vi "REPORT.DIGIAL offset.vi"(9 "Vasic":i32, 10 "Config Test IN":T1={"Config HW"={"VISA Rigol DP832"="USB0::0x1AB1::0x0E11::DP8C191500901::INSTR", "Config Rigol DP832"=[{"Channel"=0, "V Limit"=5.5, "I Limit"=0.5, "V Out"=5.0}, {"Channel"=1, "V Limit"=5.5, "I Limit"=0.8, "V Out"=5.0}, {"Channel"=2, "V Limit"=5.5, "I Limit"=0.2, "V Out"=0.0}], "CTA Test#"="CTA013 A", "FT_Handle"=432866568, "Espera acceso FT"=10, "VISA Tek MDO3104"="Rigol_DP832", "VISA Key 81160A"="Rigol_DP832"}, "Config Test"=[{"Vasic"=2.8, "Global Reset"=FALSE, "Test Register?"=FALSE, "Test ADC?"=FALSE, "Test ADC"={"Repeats ADC"=100, "Max Desviation"=0.1}, "Limits ADC"={"Low"=[1.9, 1.3, 0.65, 0.0, 1.6, 1.4, 1.4, 0.9, 2.1, 0.85, 1.9], "High"=[2.1, 1.5, 0.85, 0.1, 1.4, 1.2, 1.2, 0.7, 1.9, 0.65, 1.7]}, "Test Max PN Min NP?"=FALSE, "Limits Max PN Min NP"={"Max P Upper"=2.177000045776367, "Min P Upper"=1.474, "Max N Upper"=1.475, "Min N Upper"=0.818, "Max P Lower"=1.888, "Min P Lower "=1.321, "Max N Lower"=1.322, "Min N Lower"=0.73}, "Test Rate Scan?"=FALSE, "Vin Rate Scan"=[], "Limits Rate Scan"={"High"=[0.15, 0.242, 0.331, 0.425, 0.512, 0.6, 0.688, 0.774, 0.847, 0.91], "Low"=[0.021, 0.11, 0.189, 0.27, 0.347, 0.421, 0.487, 0.551, 0.601, 0.635]}, "Test Rate Scan Adders?"=FALSE, "Vin Rate Adders"=[], "Limits Rate Scan adders"={"High"=[], "Low"=[]}, "Test offset analog?"=FALSE, "Lim Offset Analog"={"Max Analog"=0.05, "Min Analog"=-0.05}, "Test offset digital?"=FALSE, "Lim offset Dig"={"Max Dig"=0.05}, "Vasic real f.a."=2.8, "IBIAS"=FALSE, "VALUE IBIAS"=63}, {"Vasic"=2.8, "Global Reset"=FALSE, "Test Register?"=FALSE, "Test ADC?"=FALSE, "Test ADC"={"Repeats ADC"=100, "Max Desviation"=0.1}, "Limits ADC"={"Low"=[1.9, 1.3, 0.65, 0.0, 1.6, 1.4, 1.4, 0.9, 2.1, 0.85, 1.9], "High"=[2.1, 1.5, 0.85, 0.1, 1.4, 1.2, 1.2, 0.7, 1.9, 0.65, 1.7]}, "Test Max PN Min NP?"=FALSE, "Limits Max PN Min NP"={"Max P Upper"=2.177000045776367, "Min P Upper"=1.474, "Max N Upper"=1.475, "Min N Upper"=0.818, "Max P Lower"=1.888, "Min P Lower "=1.321, "Max N Lower"=1.322, "Min N Lower"=0.73}, "Test Rate Scan?"=FALSE, "Vin Rate Scan"=[], "Limits Rate Scan"={"High"=[0.15, 0.242, 0.331, 0.425, 0.512, 0.6, 0.688, 0.774, 0.847, 0.91], "Low"=[0.021, 0.11, 0.189, 0.27, 0.347, 0.421, 0.487, 0.551, 0.601, 0.635]}, "Test Rate Scan Adders?"=FALSE, "Vin Rate Adders"=[], "Limits Rate Scan adders"={"High"=[], "Low"=[]}, "Test offset analog?"=FALSE, "Lim Offset Analog"={"Max Analog"=0.05, "Min Analog"=-0.05}, "Test offset digital?"=FALSE, "Lim offset Dig"={"Max Dig"=0.05}, "Vasic real f.a."=2.8, "IBIAS"=FALSE, "VALUE IBIAS"=63}, {"Vasic"=2.8, "Global Reset"=FALSE, "Test Register?"=FALSE, "Test ADC?"=FALSE, "Test ADC"={"Repeats ADC"=100, "Max Desviation"=0.1}, "Limits ADC"={"Low"=[1.9, 1.3, 0.65, 0.0, 1.6, 1.4, 1.4, 0.9, 2.1, 0.85, 1.9], "High"=[2.1, 1.5, 0.85, 0.1, 1.4, 1.2, 1.2, 0.7, 1.9, 0.65, 1.7]}, "Test Max PN Min NP?"=FALSE, "Limits Max PN Min NP"={"Max P Upper"=2.177000045776367, "Min P Upper"=1.474, "Max N Upper"=1.475, "Min N Upper"=0.818, "Max P Lower"=1.888, "Min P Lower "=1.321, "Max N Lower"=1.322, "Min N Lower"=0.73}, "Test Rate Scan?"=FALSE, "Vin Rate Scan"=[], "Limits Rate Scan"={"High"=[0.15, 0.242, 0.331, 0.425, 0.512, 0.6, 0.688, 0.774, 0.847, 0.91], "Low"=[0.021, 0.11, 0.189, 0.27, 0.347, 0.421, 0.487, 0.551, 0.601, 0.635]}, "Test Rate Scan Adders?"=FALSE, "Vin Rate Adders"=[], "Limits Rate Scan adders"={"High"=[], "Low"=[]}, "Test offset analog?"=FALSE, "Lim Offset Analog"={"Max Analog"=0.05, "Min Analog"=-0.05}, "Test offset digital?"=FALSE, "Lim offset Dig"={"Max Dig"=0.05}, "Vasic real f.a."=2.8, "IBIAS"=FALSE, "VALUE IBIAS"=63}, {"Vasic"=2.8, "Global Reset"=FALSE, "Test Register?"=FALSE, "Test ADC?"=FALSE, "Test ADC"={"Repeats ADC"=100, "Max Desviation"=0.1}, "Limits ADC"={"Low"=[1.9, 1.3, 0.65, 0.0, 1.6, 1.4, 1.4, 0.9, 2.1, 0.85, 1.9], "High"=[2.1, 1.5, 0.85, 0.1, 1.4, 1.2, 1.2, 0.7, 1.9, 0.65, 1.7]}, "Test Max PN Min NP?"=FALSE, "Limits Max PN Min NP"={"Max P Upper"=2.177000045776367, "Min P Upper"=1.474, "Max N Upper"=1.475, "Min N Upper"=0.818, "Max P Lower"=1.888, "Min P Lower "=1.321, "Max N Lower"=1.322, "Min N Lower"=0.73}, "Test Rate Scan?"=FALSE, "Vin Rate Scan"=[], "Limits Rate Scan"={"High"=[0.15, 0.242, 0.331, 0.425, 0.512, 0.6, 0.688, 0.774, 0.847, 0.91], "Low"=[0.021, 0.11, 0.189, 0.27, 0.347, 0.421, 0.487, 0.551, 0.601, 0.635]}, "Test Rate Scan Adders?"=FALSE, "Vin Rate Adders"=[], "Limits Rate Scan adders"={"High"=[], "Low"=[]}, "Test offset analog?"=FALSE, "Lim Offset Analog"={"Max Analog"=0.05, "Min Analog"=-0.05}, "Test offset digital?"=FALSE, "Lim offset Dig"={"Max Dig"=0.05}, "Vasic real f.a."=2.8, "IBIAS"=FALSE, "VALUE IBIAS"=63}], "Result"=[{"Vasic Volt"=0, "Test Registros"={"Default Register OK"=FALSE, "Pattern Default"=[], "Read Default"=[], "W/R Register OK"=FALSE, "Pattern W/R"=[], "Read W/R"=[]}, "Test Dacs"={"Desviacion OK"=FALSE, "Means"=[], "Deviations"=[], "Desviations OK"=[], "Means OK"=[], "Graph Histogram"=[]}, "Test Max-Min PN"={"Max P Mini N OK"=FALSE, "PTHT Max P Min N"=[], "PTHT Max P Min N OK"=[], "NTHT Max P Min N"=[], "NTHT Max P Min N OK"=[], "Min P Max N OK"=FALSE, "PTHT Max N Min P"=[], "PTHT Max N Min P OK"=[], "NTHT Max N Min P"=[], "NTHT Max N Min P OK"=[], "Ref"=[]}, "Test Rate Scan"={"Rate Scan OK"=FALSE, "DAC TH0,TH1,TH2"=[], "Volt HLTH"=[], "Rate HLTH OK"=[], "DAC TH3,TH4,TH5"=[], "Volt LLTH"=[], "Rate LLTH 2 OK"=[], "Scaler 0"=[], "Ref"=[], "OFFSET HLTH"=[], "OFFSET LLTH"=[], "Real Voltage"=[]}, "Test Rate Scan adders"={"Rate Scan Adders OK"=FALSE, "DAC TH0,TH1,TH2"=[], "Volt HLTH"=[], "Add HLTH OK"=[], "DAC TH3,TH4,TH5"=[], "Volt LLTH"=[], "Add LLTH 2 OK"=[], "Scaler 0"=[], "Ref"=[], "OFFSET HLTH"=[], "OFFSET LLTH"=[], "Real Voltage"=[]}, "Test Offset Analog"={"Offset Analog OK"=FALSE, "V ADDOUT"=[], "Offset OK"=[], "Ref"=[]}, "Test Offset Digital"={"Offset Digital OK"=FALSE, "SCALER 1 START"=[], "SCALER 1 STOP"=[], "THX START"=[], "THX STOP"=[], "VHLTH START"=[], "VHLTH STOP"=[], "Index 1 Start"=[], "index 1 Stop"=[], "SCALER 2 START"=[], "SCALER 2 STOP"=[], "THX+3 START"=[], "THX+3 STOP"=[], "VLLTH START"=[], "VLLTH STOP"=[], "Index 2 Start"=[], "index 2 Stop"=[], "Dig HLTH OK"=[], "Dig LLTH 2 OK"=[], "Ref"=[]}, "info hardware"={"Iout V1"=0.0, "Iout V2"=0.0, "Iout V3"=0.0, "Vout V1"=0.0, "Vout V2"=0.0, "Vout V3"=0.0, "Temp"=0.0}, "Test Offset Analog add"={"Offset Analog add OK"=FALSE, "V ADDOUT add"=[], "Offset add OK"=[], "Ref add"=[]}, "info temp"={"T Asic Registers"=0.0, "T Board Test. ADC"=0.0, "T Asic Max Min N P"=0.0, "T Adc count"=0.0, "T Asic Digital Offset"=0.0, "T Asic Analog Offset"=0.0, "T Asic Analog add"=0.0, "T Asic Rate Scan"=0.0, "T Asic Rate Scan Adders"=0.0, "T Final"=0.0}}, {"Vasic Volt"=0, "Test Registros"={"Default Register OK"=FALSE, "Pattern Default"=[], "Read Default"=[], "W/R Register OK"=FALSE, "Pattern W/R"=[], "Read W/R"=[]}, "Test Dacs"={"Desviacion OK"=FALSE, "Means"=[], "Deviations"=[], "Desviations OK"=[], "Means OK"=[], "Graph Histogram"=[]}, "Test Max-Min PN"={"Max P Mini N OK"=FALSE, "PTHT Max P Min N"=[], "PTHT Max P Min N OK"=[], "NTHT Max P Min N"=[], "NTHT Max P Min N OK"=[], "Min P Max N OK"=FALSE, "PTHT Max N Min P"=[], "PTHT Max N Min P OK"=[], "NTHT Max N Min P"=[], "NTHT Max N Min P OK"=[], "Ref"=[]}, "Test Rate Scan"={"Rate Scan OK"=FALSE, "DAC TH0,TH1,TH2"=[], "Volt HLTH"=[], "Rate HLTH OK"=[], "DAC TH3,TH4,TH5"=[], "Volt LLTH"=[], "Rate LLTH 2 OK"=[], "Scaler 0"=[], "Ref"=[], "OFFSET HLTH"=[], "OFFSET LLTH"=[], "Real Voltage"=[]}, "Test Rate Scan adders"={"Rate Scan Adders OK"=FALSE, "DAC TH0,TH1,TH2"=[], "Volt HLTH"=[], "Add HLTH OK"=[], "DAC TH3,TH4,TH5"=[], "Volt LLTH"=[], "Add LLTH 2 OK"=[], "Scaler 0"=[], "Ref"=[], "OFFSET HLTH"=[], "OFFSET LLTH"=[], "Real Voltage"=[]}, "Test Offset Analog"={"Offset Analog OK"=FALSE, "V ADDOUT"=[], "Offset OK"=[], "Ref"=[]}, "Test Offset Digital"={"Offset Digital OK"=FALSE, "SCALER 1 START"=[], "SCALER 1 STOP"=[], "THX START"=[], "THX STOP"=[], "VHLTH START"=[], "VHLTH STOP"=[], "Index 1 Start"=[], "index 1 Stop"=[], "SCALER 2 START"=[], "SCALER 2 STOP"=[], "THX+3 START"=[], "THX+3 STOP"=[], "VLLTH START"=[], "VLLTH STOP"=[], "Index 2 Start"=[], "index 2 Stop"=[], "Dig HLTH OK"=[], "Dig LLTH 2 OK"=[], "Ref"=[]}, "info hardware"={"Iout V1"=0.0, "Iout V2"=0.0, "Iout V3"=0.0, "Vout V1"=0.0, "Vout V2"=0.0, "Vout V3"=0.0, "Temp"=0.0}, "Test Offset Analog add"={"Offset Analog add OK"=FALSE, "V ADDOUT add"=[], "Offset add OK"=[], "Ref add"=[]}, "info temp"={"T Asic Registers"=0.0, "T Board Test. ADC"=0.0, "T Asic Max Min N P"=0.0, "T Adc count"=0.0, "T Asic Digital Offset"=0.0, "T Asic Analog Offset"=0.0, "T Asic Analog add"=0.0, "T Asic Rate Scan"=0.0, "T Asic Rate Scan Adders"=0.0, "T Final"=0.0}}, {"Vasic Volt"=0, "Test Registros"={"Default Register OK"=FALSE, "Pattern Default"=[], "Read Default"=[], "W/R Register OK"=FALSE, "Pattern W/R"=[], "Read W/R"=[]}, "Test Dacs"={"Desviacion OK"=FALSE, "Means"=[], "Deviations"=[], "Desviations OK"=[], "Means OK"=[], "Graph Histogram"=[]}, "Test Max-Min PN"={"Max P Mini N OK"=FALSE, "PTHT Max P Min N"=[], "PTHT Max P Min N OK"=[], "NTHT Max P Min N"=[], "NTHT Max P Min N OK"=[], "Min P Max N OK"=FALSE, "PTHT Max N Min P"=[], "PTHT Max N Min P OK"=[], "NTHT Max N Min P"=[], "NTHT Max N Min P OK"=[], "Ref"=[]}, "Test Rate Scan"={"Rate Scan OK"=FALSE, "DAC TH0,TH1,TH2"=[], "Volt HLTH"=[], "Rate HLTH OK"=[], "DAC TH3,TH4,TH5"=[], "Volt LLTH"=[], "Rate LLTH 2 OK"=[], "Scaler 0"=[], "Ref"=[], "OFFSET HLTH"=[], "OFFSET LLTH"=[], "Real Voltage"=[]}, "Test Rate Scan adders"={"Rate Scan Adders OK"=FALSE, "DAC TH0,TH1,TH2"=[], "Volt HLTH"=[], "Add HLTH OK"=[], "DAC TH3,TH4,TH5"=[], "Volt LLTH"=[], "Add LLTH 2 OK"=[], "Scaler 0"=[], "Ref"=[], "OFFSET HLTH"=[], "OFFSET LLTH"=[], "Real Voltage"=[]}, "Test Offset Analog"={"Offset Analog OK"=FALSE, "V ADDOUT"=[], "Offset OK"=[], "Ref"=[]}, "Test Offset Digital"={"Offset Digital OK"=FALSE, "SCALER 1 START"=[], "SCALER 1 STOP"=[], "THX START"=[], "THX STOP"=[], "VHLTH START"=[], "VHLTH STOP"=[], "Index 1 Start"=[], "index 1 Stop"=[], "SCALER 2 START"=[], "SCALER 2 STOP"=[], "THX+3 START"=[], "THX+3 STOP"=[], "VLLTH START"=[], "VLLTH STOP"=[], "Index 2 Start"=[], "index 2 Stop"=[], "Dig HLTH OK"=[], "Dig LLTH 2 OK"=[], "Ref"=[]}, "info hardware"={"Iout V1"=0.0, "Iout V2"=0.0, "Iout V3"=0.0, "Vout V1"=0.0, "Vout V2"=0.0, "Vout V3"=0.0, "Temp"=0.0}, "Test Offset Analog add"={"Offset Analog add OK"=FALSE, "V ADDOUT add"=[], "Offset add OK"=[], "Ref add"=[]}, "info temp"={"T Asic Registers"=0.0, "T Board Test. ADC"=0.0, "T Asic Max Min N P"=0.0, "T Adc count"=0.0, "T Asic Digital Offset"=0.0, "T Asic Analog Offset"=0.0, "T Asic Analog add"=0.0, "T Asic Rate Scan"=0.0, "T Asic Rate Scan Adders"=0.0, "T Final"=0.0}}, {"Vasic Volt"=0, "Test Registros"={"Default Register OK"=FALSE, "Pattern Default"=[], "Read Default"=[], "W/R Register OK"=FALSE, "Pattern W/R"=[], "Read W/R"=[]}, "Test Dacs"={"Desviacion OK"=FALSE, "Means"=[], "Deviations"=[], "Desviations OK"=[], "Means OK"=[], "Graph Histogram"=[]}, "Test Max-Min PN"={"Max P Mini N OK"=FALSE, "PTHT Max P Min N"=[], "PTHT Max P Min N OK"=[], "NTHT Max P Min N"=[], "NTHT Max P Min N OK"=[], "Min P Max N OK"=FALSE, "PTHT Max N Min P"=[], "PTHT Max N Min P OK"=[], "NTHT Max N Min P"=[], "NTHT Max N Min P OK"=[], "Ref"=[]}, "Test Rate Scan"={"Rate Scan OK"=FALSE, "DAC TH0,TH1,TH2"=[], "Volt HLTH"=[], "Rate HLTH OK"=[], "DAC TH3,TH4,TH5"=[], "Volt LLTH"=[], "Rate LLTH 2 OK"=[], "Scaler 0"=[], "Ref"=[], "OFFSET HLTH"=[], "OFFSET LLTH"=[], "Real Voltage"=[]}, "Test Rate Scan adders"={"Rate Scan Adders OK"=FALSE, "DAC TH0,TH1,TH2"=[], "Volt HLTH"=[], "Add HLTH OK"=[], "DAC TH3,TH4,TH5"=[], "Volt LLTH"=[], "Add LLTH 2 OK"=[], "Scaler 0"=[], "Ref"=[], "OFFSET HLTH"=[], "OFFSET LLTH"=[], "Real Voltage"=[]}, "Test Offset Analog"={"Offset Analog OK"=FALSE, "V ADDOUT"=[], "Offset OK"=[], "Ref"=[]}, "Test Offset Digital"={"Offset Digital OK"=FALSE, "SCALER 1 START"=[], "SCALER 1 STOP"=[], "THX START"=[], "THX STOP"=[], "VHLTH START"=[], "VHLTH STOP"=[], "Index 1 Start"=[], "index 1 Stop"=[], "SCALER 2 START"=[], "SCALER 2 STOP"=[], "THX+3 START"=[], "THX+3 STOP"=[], "VLLTH START"=[], "VLLTH STOP"=[], "Index 2 Start"=[], "index 2 Stop"=[], "Dig HLTH OK"=[], "Dig LLTH 2 OK"=[], "Ref"=[]}, "info hardware"={"Iout V1"=0.0, "Iout V2"=0.0, "Iout V3"=0.0, "Vout V1"=0.0, "Vout V2"=0.0, "Vout V3"=0.0, "Temp"=0.0}, "Test Offset Analog add"={"Offset Analog add OK"=FALSE, "V ADDOUT add"=[], "Offset add OK"=[], "Ref add"=[]}, "info temp"={"T Asic Registers"=0.0, "T Board Test. ADC"=0.0, "T Asic Max Min N P"=0.0, "T Adc count"=0.0, "T Asic Digital Offset"=0.0, "T Asic Analog Offset"=0.0, "T Asic Analog add"=0.0, "T Asic Rate Scan"=0.0, "T Asic Rate Scan Adders"=0.0, "T Final"=0.0}}], "Execucion Test"={"Vasic Actual"=0}, "Config VGA"={"Theoretical Voltage"=[0.1, 0.2, 0.3, 0.4, 0.5, 0.6, 0.7, 0.8, 0.9, 1.0], "Real Voltage"=[0.10285, 0.20714, 0.29957, 0.40485, 0.49571, 0.60685, 0.69771, 0.80114, 0.89714, 0.99885], "Pulse Width"=57344, "Frecuency Pulse"=1000000.0, "VGA Gain"=[9, 16, 24, 34, 43, 52, 61, 72, 81, 93]}, "Test Info"={"Asic"="", "Operator"="", "Place"="", "Time start"=timestamp(0 s since 1904-01-01), "Time stop"=timestamp(0 s since 1904-01-01)}, "Info machine"={"SO"="", "SO Name"="", "SO Ver"="", "SO Build"="", "CPU"="", "APP"="", "APP YEAR"="", "APP ver"="", "APP User"="", "APP Serail"="", "MAC"=[], "PC NAME"=[], "PC IP"=[], "BIOS MANU"="", "BIOS NAME"="", "BIOS SERIAL"="", "BOARD MANU"="", "BOARD NAME"="", "BOARD SERIAL"="", "Driver Version"="", "Library Version"="", "FPGA Ver"=0, "ID CTA board"=0, "LAST BOOT"="", "LABVIEW Ver"=0}, "Partial Report"="", "CONFIG GEN"=[]} {"CONFIG GEN"."Vasic Theorical" min=1.0 max=1000000.0 step=1.0 format="%#_6pV"; "CONFIG GEN"."Frequency" min=0.001 max=333000000.0 step=1000.0 format="%#_6pHz"; "CONFIG GEN"."Leading Edge Time" min=1e-09 max=1.0 step=1e-10 format="%#_6ps"; "CONFIG GEN"."Trailing Edge Time" min=1e-09 max=1.0 step=1e-10 format="%#_6ps"; "CONFIG GEN"."Delay" min=0.0 max=1.0 step=1e-12 format="%#_6ps"; "CONFIG GEN"."Trigger Level Sync" items=["ECL", "TTL"]; "CONFIG GEN"."Trigger Sync Out" items=["AB"=3, "B"=2, "A"=1, "None"=0]; "CONFIG GEN"."Load" min=1.0 max=1000000.0 step=1.0 format="%#_6p"; "CONFIG GEN"."DC Offset" min=-10.0 max=10.0 step=0.1 format="%#_6pV"; "CONFIG GEN"."Amplitude" min=0.05 max=5.0 step=0.001 format="%#_6pV"; "CONFIG GEN"."Width Time" min=1.5e-09 max=1.0 step=1e-10 format="%#_6ps"; "CONFIG GEN"."Channel" items=["Channel1"=1, "Channel2"=2]; "Config VGA"."Theoretical Voltage" format="%1.4f"; "Config VGA"."VGA Gain" format="%02x"; "Config VGA"."Frecuency Pulse" format="%0_2p"; "Config VGA"."Pulse Width" format="%04x"; "Config VGA"."Real Voltage" format="%1.5f"; "Config Test"."VALUE IBIAS" max=63 step=1; "Config Test"."Vasic real f.a." min=2.8 max=3.8 step=0.01 format="%.2g"; "Config Test"."Limits Rate Scan adders"."Low" format="%1.3f"; "Config Test"."Limits Rate Scan adders"."High" format="%1.3f"; "Config Test"."Limits ADC"."High" format="%1.4f"; "Config Test"."Limits ADC"."Low" format="%1.3f"; "Config Test"."Lim offset Dig"."Max Dig" format="%.3g"; "Config Test"."Lim Offset Analog"."Min Analog" format="%.3g"; "Config Test"."Lim Offset Analog"."Max Analog" format="%.3g"; "Config Test"."Limits Rate Scan"."Low" format="%1.4f"; "Config Test"."Limits Rate Scan"."High" format="%1.3f"; "Config Test"."Limits Max PN Min NP"."Min P Upper" format="%.3g"; "Config Test"."Limits Max PN Min NP"."Min P Lower" format="%.3g"; "Config Test"."Limits Max PN Min NP"."Max N Lower" format="%.3g"; "Config Test"."Limits Max PN Min NP"."Max N Upper" format="%.3g"; "Config Test"."Limits Max PN Min NP"."Min N Lower" format="%.3g"; "Config Test"."Limits Max PN Min NP"."Min N Upper" format="%.3g"; "Config Test"."Limits Max PN Min NP"."Max P Upper" format="%.3g"; "Config Test"."Limits Max PN Min NP"."Max P Lower" format="%.3g"; "Config Test"."Vasic" min=2.8 max=3.8 step=0.01 format="%.2g"; "Config HW"."Config Rigol DP832"."Channel" items=["+30V Channel 1", "+30V Channel 2", "+5V Channel 3"]; "Config HW"."Config Rigol DP832"."V Limit" format="%.1g"; "Config HW"."Config Rigol DP832"."I Limit" format="%.1g"; "Config HW"."Config Rigol DP832"."V Out" format="%.1g"; "Result"."Test Registros"."Read W/R" format="%04x"; "Result"."Test Registros"."Pattern W/R" format="%04x"; "Result"."Test Registros"."Read Default" format="%04x"; "Result"."Test Registros"."Pattern Default" format="%04x"}, 11 "Text In":string) -> (3 "Text Out":string)   [LabVIEW 2019]
uses:
  Test.ctl
  TEST.TEST CONFIG HW.ctl
  Rigol DP832/DP832_Control Channels.ctl
  TEST.TEST CONFIG TEST MATRIZ.ctl
  TEST.TEST CONFIG TEST.ctl
  TEST.TEST RESULT.ctl
  test_result fvasic.ctl
  TEST.TEST EXECUTION TEST.ctl
  TEST.TEST CONFIG VGA.ctl
  TEST.TEST TEST INFO.ctl
  TEST.TEST INFO PC.ctl
  GenPulse_configurar.ctl
panel:
  # "Modo 2\nModo 3\nModo 4\nModo 2\nModo 3\nModo 4"
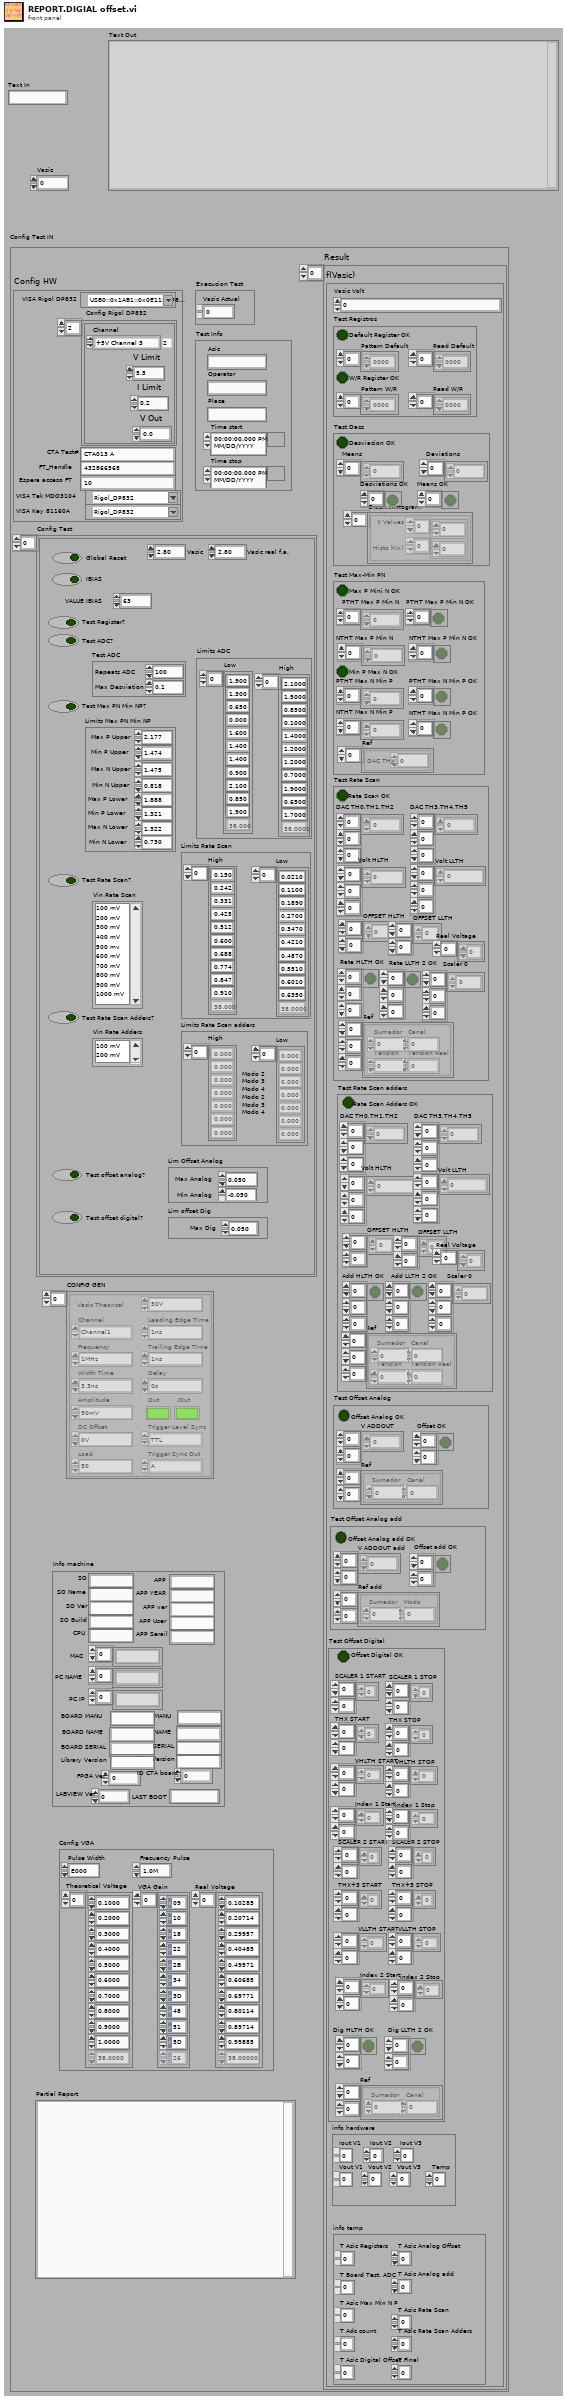
[diagram p1: front panel]
types:
  T1 = typedef "Test.ctl" = cluster{"Config HW":T2, "Config Test":T4, "Result":T6, "Execucion Test":T8, "Config VGA":T9, "Test Info":T10, "Info machine":T11, "Partial Report":string, "CONFIG GEN":T12[]}
  T2 = typedef "TEST.TEST CONFIG HW.ctl" = cluster{"VISA Rigol DP832":refnum<visa-resource-name>, "Config Rigol DP832":cluster{"Channel":T3, "V Limit":dbl, "I Limit":dbl, "V Out":dbl}[], "CTA Test#":string, "FT_Handle":u32, "Espera acceso FT":u32, "VISA Tek MDO3104":refnum<visa-resource-name>, "VISA Key 81160A":refnum<visa-resource-name>}
  T3 = typedef "DP832_Control Channels.ctl" = i32
  T4 = typedef "TEST.TEST CONFIG TEST MATRIZ.ctl" = T5[]
  T5 = typedef "TEST.TEST CONFIG TEST.ctl" = cluster{"Vasic":dbl, "Global Reset":bool, "Test Register?":bool, "Test ADC?":bool, "Test ADC":cluster{"Repeats ADC":i32, "Max Desviation":dbl}, "Limits ADC":cluster{"Low":dbl[], "High":dbl[]}, "Test Max PN Min NP?":bool, "Limits Max PN Min NP":cluster{"Max P Upper":dbl, "Min P Upper":dbl, "Max N Upper":dbl, "Min N Upper":dbl, "Max P Lower":dbl, "Min P Lower ":dbl, "Max N Lower":dbl, "Min N Lower":dbl}, "Test Rate Scan?":bool, "Vin Rate Scan":i32[], "Limits Rate Scan":cluster{"High":dbl[], "Low":dbl[]}, "Test Rate Scan Adders?":bool, "Vin Rate Adders":i32[], "Limits Rate Scan adders":cluster{"High":dbl[], "Low":dbl[]}, "Test offset analog?":bool, "Lim Offset Analog":cluster{"Max Analog":dbl, "Min Analog":dbl}, "Test offset digital?":bool, "Lim offset Dig":cluster{"Max Dig":dbl}, "Vasic real f.a.":dbl, "IBIAS":bool, "VALUE IBIAS":u8}
  T6 = typedef "TEST.TEST RESULT.ctl" = T7[]
  T7 = typedef "test_result fvasic.ctl" = cluster{"Vasic Volt":i32, "Test Registros":cluster{"Default Register OK":bool, "Pattern Default":u16[], "Read Default":u16[], "W/R Register OK":bool, "Pattern W/R":u16[], "Read W/R":u16[]}, "Test Dacs":cluster{"Desviacion OK":bool, "Means":dbl[], "Deviations":dbl[], "Desviations OK":bool[], "Means OK":bool[], "Graph Histogram":cluster{"X Values":dbl[], "Histo h(x)":i32[]}[]}, "Test Max-Min PN":cluster{"Max P Mini N OK":bool, "PTHT Max P Min N":dbl[], "PTHT Max P Min N OK":bool[], "NTHT Max P Min N":dbl[], "NTHT Max P Min N OK":bool[], "Min P Max N OK":bool, "PTHT Max N Min P":dbl[], "PTHT Max N Min P OK":bool[], "NTHT Max N Min P":dbl[], "NTHT Max N Min P OK":bool[], "Ref":cluster{"DAC THx":u8}[]}, "Test Rate Scan":cluster{"Rate Scan OK":bool, "DAC TH0,TH1,TH2":u16[][][], "Volt HLTH":dbl[][][], "Rate HLTH OK":bool[][][], "DAC TH3,TH4,TH5":u16[][][], "Volt LLTH":dbl[][][], "Rate LLTH 2 OK":bool[][][], "Scaler 0":u16[][][], "Ref":cluster{"Sumador":u8, "Canal":u8, "Tension":u8, "Tension Real":dbl}[][][], "OFFSET HLTH":dbl[][], "OFFSET LLTH":dbl[][], "Real Voltage":dbl[]}, "Test Rate Scan adders":cluster{"Rate Scan Adders OK":bool, "DAC TH0,TH1,TH2":u16[][][], "Volt HLTH":dbl[][][], "Add HLTH OK":bool[][][], "DAC TH3,TH4,TH5":u16[][][], "Volt LLTH":dbl[][][], "Add LLTH 2 OK":bool[][][], "Scaler 0":u16[][][], "Ref":cluster{"Sumador":u8, "Canal":u8, "Tension":u8, "Tension Real":dbl}[][][], "OFFSET HLTH":dbl[][], "OFFSET LLTH":dbl[][], "Real Voltage":dbl[]}, "Test Offset Analog":cluster{"Offset Analog OK":bool, "V ADDOUT":dbl[][], "Offset OK":bool[][], "Ref":cluster{"Sumador":u8, "Canal":u8}[][]}, "Test Offset Digital":cluster{"Offset Digital OK":bool, "SCALER 1 START":u16[][], "SCALER 1 STOP":u16[][], "THX START":u16[][], "THX STOP":u16[][], "VHLTH START":dbl[][], "VHLTH STOP":dbl[][], "Index 1 Start":i32[][], "index 1 Stop":i32[][], "SCALER 2 START":u16[][], "SCALER 2 STOP":u16[][], "THX+3 START":u16[][], "THX+3 STOP":u16[][], "VLLTH START":dbl[][], "VLLTH STOP":dbl[][], "Index 2 Start":i32[][], "index 2 Stop":i32[][], "Dig HLTH OK":bool[][], "Dig LLTH 2 OK":bool[][], "Ref":cluster{"Sumador":u8, "Canal":u8}[][]}, "info hardware":cluster{"Iout V1":dbl, "Iout V2":dbl, "Iout V3":dbl, "Vout V1":dbl, "Vout V2":dbl, "Vout V3":dbl, "Temp":dbl}, "Test Offset Analog add":cluster{"Offset Analog add OK":bool, "V ADDOUT add":dbl[][], "Offset add OK":bool[][], "Ref add":cluster{"Sumador":u8, "Modo":u8}[][]}, "info temp":cluster{"T Asic Registers":dbl, "T Board Test. ADC":dbl, "T Asic Max Min N P":dbl, "T Adc count":dbl, "T Asic Digital Offset":dbl, "T Asic Analog Offset":dbl, "T Asic Analog add":dbl, "T Asic Rate Scan":dbl, "T Asic Rate Scan Adders":dbl, "T Final":dbl}}
  T8 = typedef "TEST.TEST EXECUTION TEST.ctl" = cluster{"Vasic Actual":i32}
  T9 = typedef "TEST.TEST CONFIG VGA.ctl" = cluster{"Theoretical Voltage":dbl[], "Real Voltage":dbl[], "Pulse Width":u16, "Frecuency Pulse":dbl, "VGA Gain":u8[]}
  T10 = typedef "TEST.TEST TEST INFO.ctl" = cluster{"Asic":string, "Operator":string, "Place":string, "Time start":timestamp, "Time stop":timestamp}
  T11 = typedef "TEST.TEST INFO PC.ctl" = cluster{"SO":string, "SO Name":string, "SO Ver":string, "SO Build":string, "CPU":string, "APP":string, "APP YEAR":string, "APP ver":string, "APP User":string, "APP Serail":string, "MAC":string[], "PC NAME":string[], "PC IP":string[], "BIOS MANU":string, "BIOS NAME":string, "BIOS SERIAL":string, "BOARD MANU":string, "BOARD NAME":string, "BOARD SERIAL":string, "Driver Version":string, "Library Version":string, "FPGA Ver":u8, "ID CTA board":u64, "LAST BOOT":string, "LABVIEW Ver":u32}
  T12 = typedef "GenPulse_configurar.ctl" = cluster{"Channel":u16, "Frequency":dbl, "Width Time":dbl, "Amplitude":dbl, "DC Offset":dbl, "Load":dbl, "Leading Edge Time":dbl, "Trailing Edge Time":dbl, "Delay":dbl, "Out":bool, "/Out":bool, "Trigger Level Sync":u16, "Trigger Sync Out":u16, "Vasic Theorical":dbl}
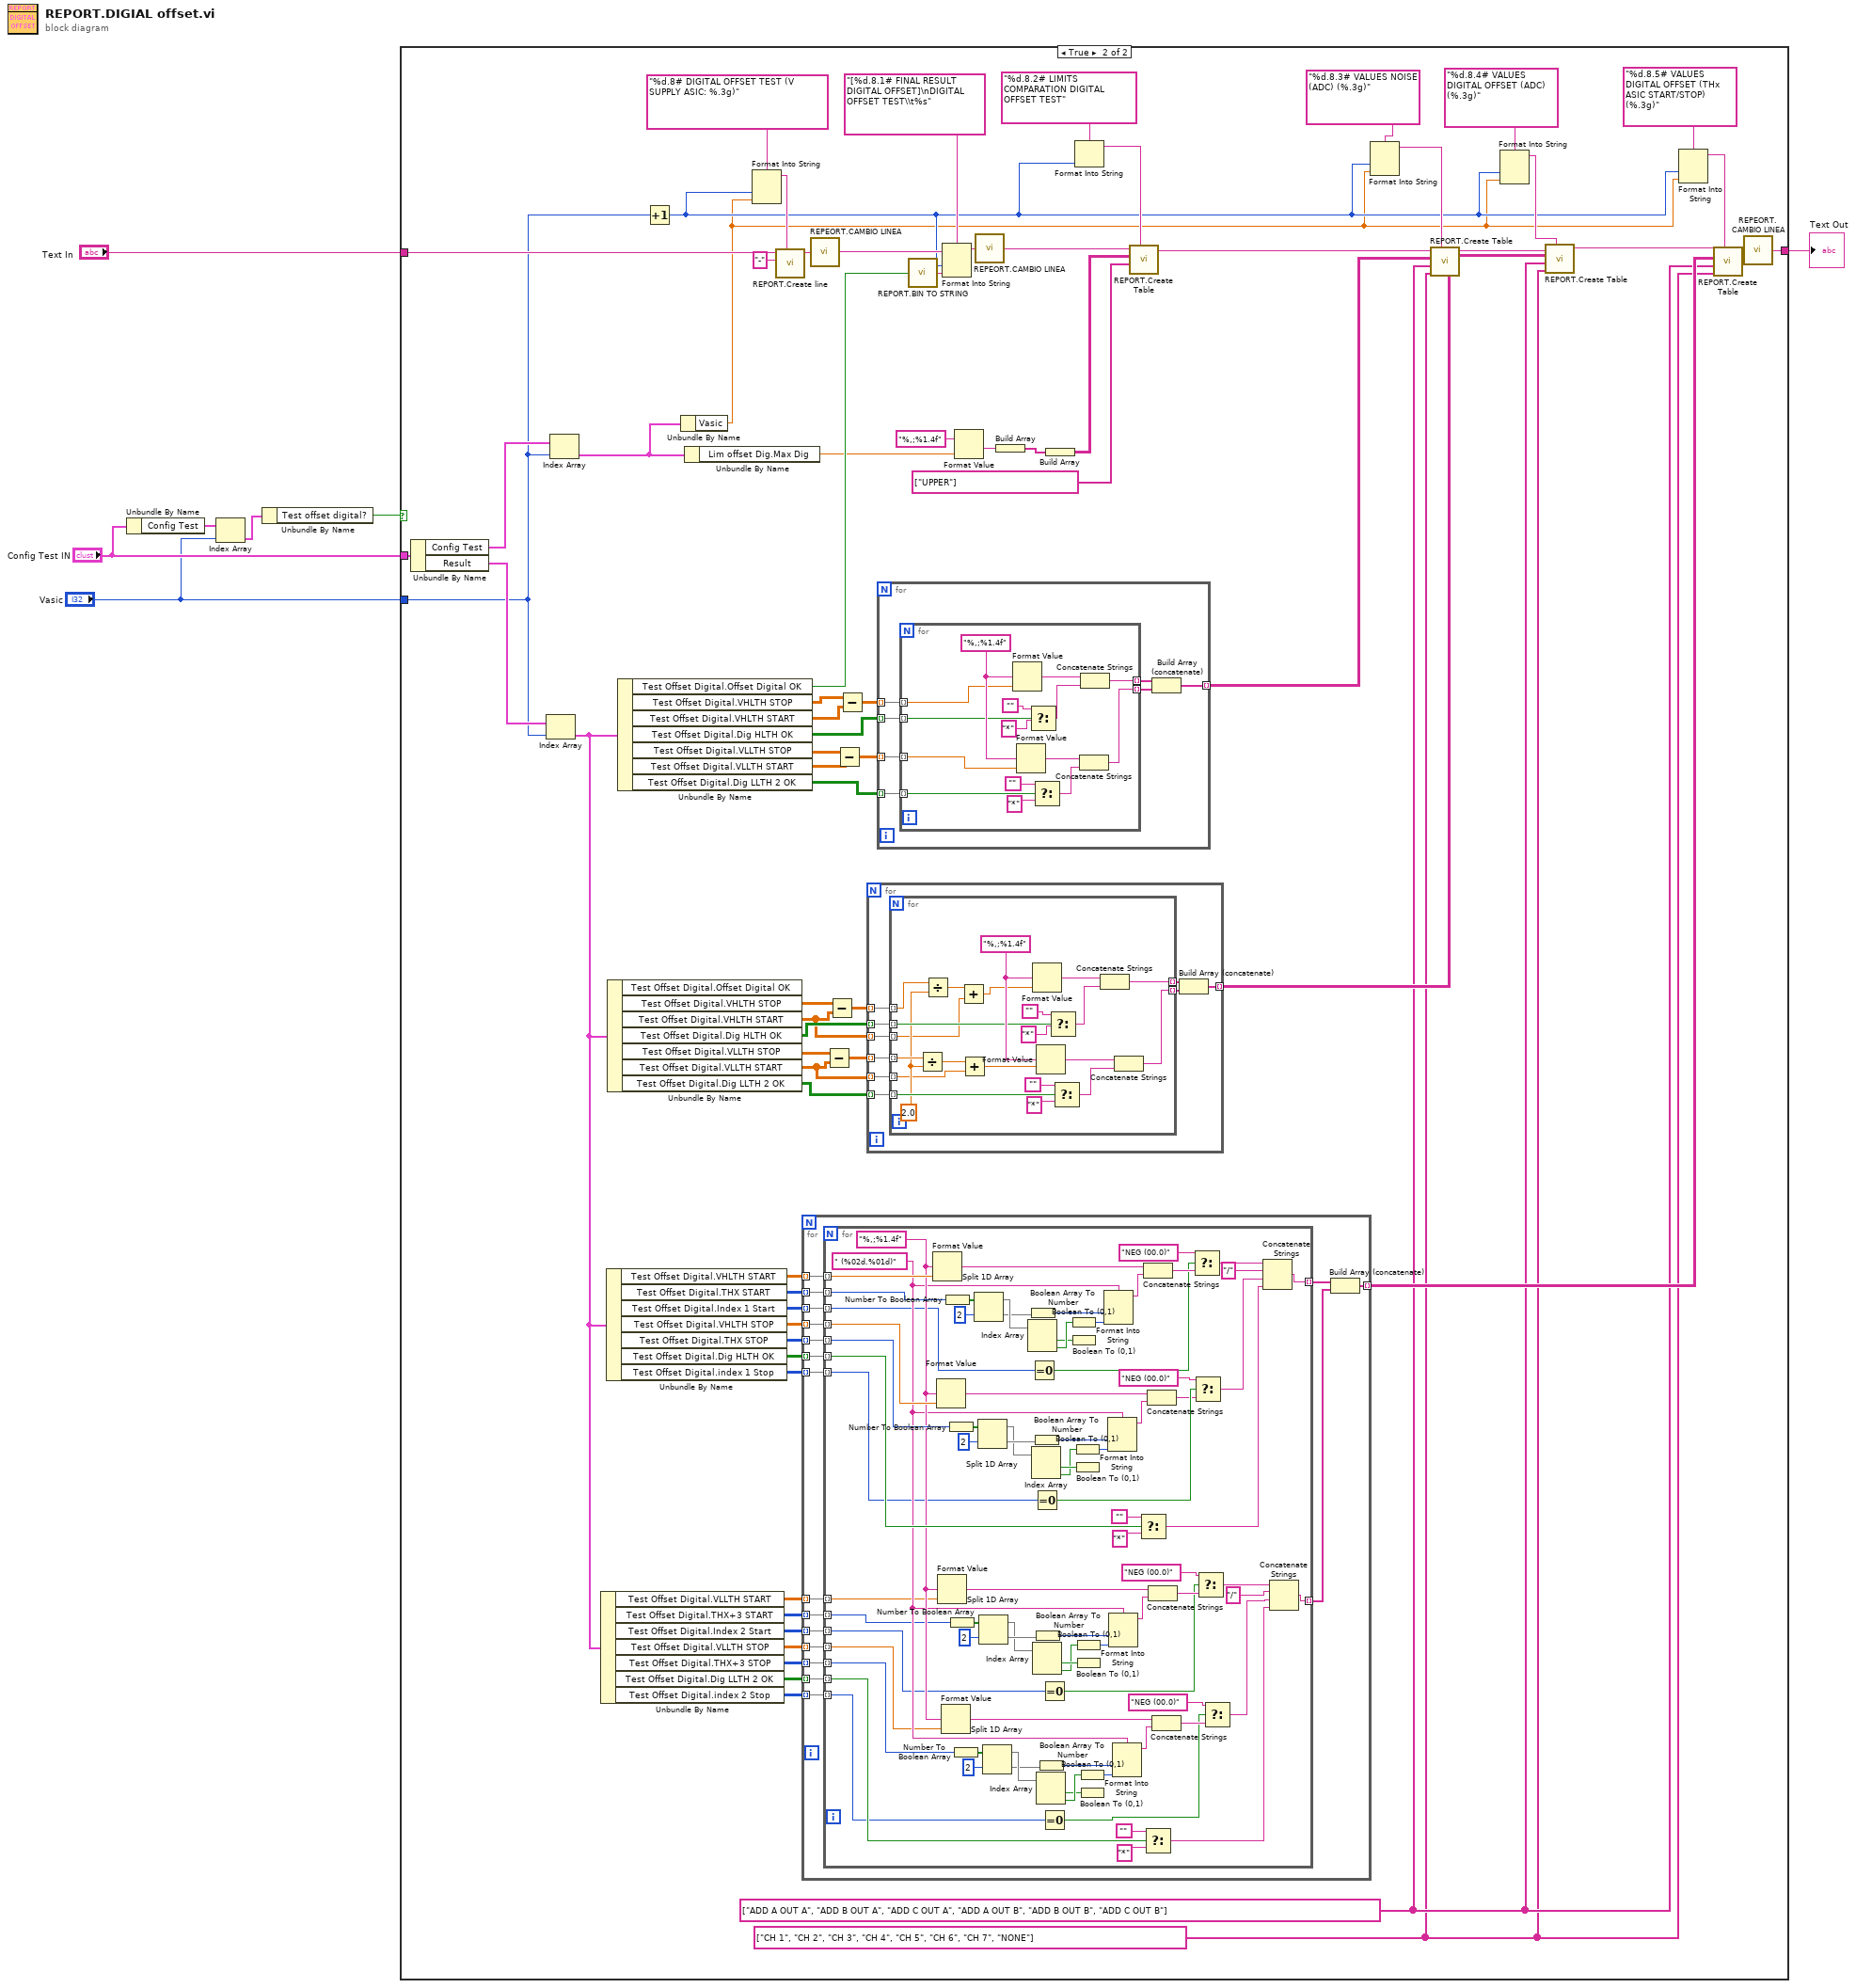
[diagram p0: block diagram]
diagram:
  n1 = Unbundle By Name("Config Test IN") -> ("Config Test"=w5:T4)
  n2 = Index Array(array=w5, index="Vasic") -> (element=w4:T5)
  n3 = Unbundle By Name(w4) -> ("Test offset digital?"=w1:bool)
  n4 = case shown="True" w1 {
    tunnel: "Text In" -> [w8 w81]
    tunnel: [w8 w80] -> w6
    tunnel: "Config Test IN" -> [_ w28]
    tunnel: "Vasic" -> [_ w27]
    frame False {
    }
    frame True {
      w13 = string[] ["CH 1", "CH 2", "CH 3", "CH 4", "CH 5", "CH 6", "CH 7", "NONE"] ("Row Headers")
      w14 = string[] ["ADD A OUT A", "ADD B OUT A", "ADD C OUT A", "ADD A OUT B", "ADD B OUT B", "ADD C OUT B"] ("Column Headers")
      n5 = Unbundle By Name(w28) -> ("Config Test"=w78:T4, "Result"=w79:T6)
      n6 = Index Array(array=w79, index=w27) -> (element=w18:T7)
      n7 = Index Array(array=w78, index=w27) -> (element=w40:T5)
      n8 = Unbundle By Name(w18) -> ("Test Offset Digital.VLLTH START"=w47:dbl[][], "Test Offset Digital.THX+3 START"=w48:u16[][], "Test Offset Digital.Index 2 Start"=w44:i32[][], "Test Offset Digital.VLLTH STOP"=w49:dbl[][], "Test Offset Digital.THX+3 STOP"=w50:u16[][], "Test Offset Digital.Dig LLTH 2 OK"=w51:bool[][], "Test Offset Digital.index 2 Stop"=w43:i32[][])
      n9 = Unbundle By Name(w18) -> ("Test Offset Digital.VHLTH START"=w56:dbl[][], "Test Offset Digital.THX START"=w55:u16[][], "Test Offset Digital.Index 1 Start"=w45:i32[][], "Test Offset Digital.VHLTH STOP"=w53:dbl[][], "Test Offset Digital.THX STOP"=w52:u16[][], "Test Offset Digital.Dig HLTH OK"=w54:bool[][], "Test Offset Digital.index 1 Stop"=w46:i32[][])
      n10 = Unbundle By Name(w18) -> ("Test Offset Digital.VHLTH STOP"=w16:dbl[][], "Test Offset Digital.VHLTH START"=w10:dbl[][], "Test Offset Digital.Dig HLTH OK"=w20:bool[][], "Test Offset Digital.VLLTH STOP"=w17:dbl[][], "Test Offset Digital.VLLTH START"=w11:dbl[][], "Test Offset Digital.Dig LLTH 2 OK"=w21:bool[][])  [unwired: 1 out]
      n11 = Unbundle By Name(w18) -> ("Test Offset Digital.Offset Digital OK"=w77:bool, "Test Offset Digital.VHLTH STOP"=w67:dbl[][], "Test Offset Digital.VHLTH START"=w66:dbl[][], "Test Offset Digital.Dig HLTH OK"=w62:bool[][], "Test Offset Digital.VLLTH STOP"=w64:dbl[][], "Test Offset Digital.VLLTH START"=w63:dbl[][], "Test Offset Digital.Dig LLTH 2 OK"=w61:bool[][])
      n12 = Increment(x=w27) -> (x+1=w12:i32)
      n13 = Unbundle By Name(w40) -> ("Vasic"=w9:dbl)
      n14 = Unbundle By Name(w40) -> ("Lim offset Dig.Max Dig"=w68:dbl)
      n15 = Format Into String(format string="%d.8# DIGITAL OFFSET TEST (V SUPPLY ASIC: %.3g)" ("Secction"), w12, w9) -> (resulting string=w38:string)  [unwired: 2 in, 1 out]
      n16 = call "REPORT.Create line.vi"("Secction"=w38, "Char"="-", "Text In"=w81) -> ("Text Out"=w42:string)  [unwired: 8 in]
      n17 = for {
        tunnel: w56 -> [w129] mode=indexing
        tunnel: w55 -> [w128] mode=indexing
        tunnel: [w125] -> w58 mode=indexing
        tunnel: w54 -> [w124] mode=indexing
        tunnel: w53 -> [w123] mode=indexing
        tunnel: w52 -> [w122] mode=indexing
        tunnel: w47 -> [w121] mode=indexing
        tunnel: w48 -> [w120] mode=indexing
        tunnel: w49 -> [w119] mode=indexing
        tunnel: w50 -> [w118] mode=indexing
        tunnel: w51 -> [w117] mode=indexing
        tunnel: w46 -> [w116] mode=indexing
        tunnel: w45 -> [w115] mode=indexing
        tunnel: w44 -> [w114] mode=indexing
        tunnel: w43 -> [w113] mode=indexing
        n18 = for {
          tunnel: w129 -> [w211] mode=indexing
          tunnel: w128 -> [w197] mode=indexing
          tunnel: [w206] -> w127 mode=indexing
          tunnel: [w152] -> w126 mode=indexing
          tunnel: w124 -> [w209] mode=indexing
          tunnel: w123 -> [w184] mode=indexing
          tunnel: w122 -> [w183] mode=indexing
          tunnel: w121 -> [w157] mode=indexing
          tunnel: w120 -> [w156] mode=indexing
          tunnel: w119 -> [w155] mode=indexing
          tunnel: w118 -> [w154] mode=indexing
          tunnel: w117 -> [w153] mode=indexing
          tunnel: w116 -> [w145] mode=indexing
          tunnel: w115 -> [w151] mode=indexing
          tunnel: w114 -> [w136] mode=indexing
          tunnel: w113 -> [w131] mode=indexing
          w158 = " (%02d.%01d)" ("format string")
          w159 = "%,;%1.4f" ("format string")
          n19 = Format Value(format string=w159, value (0)=w211) -> (output string=w210:string)  [unwired: 1 in]
          n20 = Format Value(format string=w159, value (0)=w184) -> (output string=w186:string)  [unwired: 1 in]
          n21 = Format Value(format string=w159, value (0)=w157) -> (output string=w160:string)  [unwired: 1 in]
          n22 = Format Value(format string=w159, value (0)=w155) -> (output string=w181:string)  [unwired: 1 in]
          n23 = Number To Boolean Array(number=w197) -> (Boolean array=w198:bool[])
          n24 = Number To Boolean Array(number=w183) -> (Boolean array=w194:bool[])
          n25 = Number To Boolean Array(number=w156) -> (Boolean array=w170:bool[])
          n26 = Number To Boolean Array(number=w154) -> (Boolean array=w173:bool[])
          n27 = Split 1D Array(array=w198, index=2) -> (first subarray=w202:bool[], second subarray=w201:bool[])
          n28 = Split 1D Array(array=w194, index=2) -> (first subarray=w190:bool[], second subarray=w191:bool[])
          n29 = Split 1D Array(array=w170, index=2) -> (first subarray=w166:bool[], second subarray=w167:bool[])
          n30 = Split 1D Array(array=w173, index=2) -> (first subarray=w177:bool[], second subarray=w176:bool[])
          n31 = Index Array(array=w202) -> (element #1=w203:bool, element #2=w205:bool)  [unwired: 2 in]
          n32 = Boolean Array To Number(Boolean array=w201) -> (number=w200:u32)
          n33 = Equal To 0?(x=w151) -> (x = 0?=w149:bool)
          n34 = Index Array(array=w190) -> (element #1=w189:bool, element #2=w187:bool)  [unwired: 2 in]
          n35 = Boolean Array To Number(Boolean array=w191) -> (number=w192:u32)
          n36 = Equal To 0?(x=w145) -> (x = 0?=w144:bool)
          n37 = Index Array(array=w166) -> (element #1=w165:bool, element #2=w163:bool)  [unwired: 2 in]
          n38 = Boolean Array To Number(Boolean array=w167) -> (number=w168:u32)
          n39 = Index Array(array=w177) -> (element #1=w178:bool, element #2=w180:bool)  [unwired: 2 in]
          n40 = Boolean Array To Number(Boolean array=w176) -> (number=w175:u32)
          n41 = Equal To 0?(x=w136) -> (x = 0?=w135:bool)
          n42 = Equal To 0?(x=w131) -> (x = 0?=w130:bool)
          n43 = Boolean To (0,1)(Boolean=w205) -> (0, 1=w204:i16)
          n44 = Boolean To (0,1)(Boolean=w203) -> ()  [unwired: 1 out]
          n45 = Boolean To (0,1)(Boolean=w187) -> (0, 1=w188:i16)
          n46 = Boolean To (0,1)(Boolean=w189) -> ()  [unwired: 1 out]
          n47 = Boolean To (0,1)(Boolean=w163) -> (0, 1=w164:i16)
          n48 = Boolean To (0,1)(Boolean=w165) -> ()  [unwired: 1 out]
          n49 = Boolean To (0,1)(Boolean=w180) -> (0, 1=w179:i16)
          n50 = Boolean To (0,1)(Boolean=w178) -> ()  [unwired: 1 out]
          n51 = Format Into String(format string=w158, w200, w204) -> (resulting string=w196:string)  [unwired: 2 in, 1 out]
          n52 = Format Into String(format string=w158, w192, w188) -> (resulting string=w195:string)  [unwired: 2 in, 1 out]
          n53 = Format Into String(format string=w158, w168, w164) -> (resulting string=w171:string)  [unwired: 2 in, 1 out]
          n54 = Format Into String(format string=w158, w175, w179) -> (resulting string=w172:string)  [unwired: 2 in, 1 out]
          n55 = Select(t="", s=w209, f="*") -> (s? t:f=w185:string)
          n56 = Concatenate Strings(w210, w196) -> (w150:string)
          n57 = Select(t="", s=w153, f="*") -> (s? t:f=w182:string)
          n58 = Concatenate Strings(w186, w195) -> (w142:string)
          n59 = Concatenate Strings(w160, w171) -> (w137:string)
          n60 = Concatenate Strings(w181, w172) -> (w140:string)
          n61 = Select(t="NEG (00.0)", s=w149, f=w150) -> (s? t:f=w147:string)
          n62 = Select(t="NEG (00.0)", s=w144, f=w142) -> (s? t:f=w141:string)
          n63 = Select(t="NEG (00.0)", s=w135, f=w137) -> (s? t:f=w134:string)
          n64 = Select(t="NEG (00.0)", s=w130, f=w140) -> (s? t:f=w132:string)
          n65 = Concatenate Strings(w147, "/" ("string"), w141, w185) -> (w206:string)
          n66 = Concatenate Strings(w134, "/" ("string"), w132, w182) -> (w152:string)
        }
        n67 = Build Array (concatenate)(w127, w126) -> (w125:string[])
      }
      n68 = call "REPEORT.CAMBIO LINEA.vi"("Text Out"=w42) -> ("String"=w41:string)  [unwired: 8 in]
      n69 = Subtract(x=w17, y=w11) -> (x-y=w22:dbl[][])
      n70 = Subtract(x=w16, y=w10) -> (x-y=w19:dbl[][])
      n71 = Subtract(x=w64, y=w63) -> (x-y=w60:dbl[][])
      n72 = Subtract(x=w67, y=w66) -> (x-y=w65:dbl[][])
      n73 = for {
        tunnel: w19 -> [w90] mode=indexing
        tunnel: w20 -> [w89] mode=indexing
        tunnel: w22 -> [w88] mode=indexing
        tunnel: w21 -> [w87] mode=indexing
        tunnel: [w84] -> w15 mode=indexing
        tunnel: w11 -> [w83] mode=indexing
        tunnel: w10 -> [w82] mode=indexing
        n74 = for {
          tunnel: w90 -> [w99] mode=indexing
          tunnel: w89 -> [w101] mode=indexing
          tunnel: w88 -> [w98] mode=indexing
          tunnel: w87 -> [w100] mode=indexing
          tunnel: [w108] -> w86 mode=indexing
          tunnel: [w104] -> w85 mode=indexing
          tunnel: w83 -> [w94] mode=indexing
          tunnel: w82 -> [w93] mode=indexing
          w97 = 2.0 ("y")
          w112 = "%,;%1.4f" ("format string")
          n75 = Divide(x=w98, y=w97) -> (x/y=w95:dbl)
          n76 = Divide(x=w99, y=w97) -> (x/y=w96:dbl)
          n77 = Add(x=w96, y=w93) -> (x+y=w92:dbl)
          n78 = Add(x=w95, y=w94) -> (x+y=w91:dbl)
          n79 = Format Value(format string=w112, value (0)=w92) -> (output string=w103:string)  [unwired: 1 in]
          n80 = Format Value(format string=w112, value (0)=w91) -> (output string=w102:string)  [unwired: 1 in]
          n81 = Select(t="", s=w101, f="*") -> (s? t:f=w109:string)
          n82 = Select(t="", s=w100, f="*") -> (s? t:f=w105:string)
          n83 = Concatenate Strings(w103, w109) -> (w108:string)
          n84 = Concatenate Strings(w102, w105) -> (w104:string)
        }
        n85 = Build Array (concatenate)(w86, w85) -> (w84:string[])
      }
      n86 = for {
        tunnel: w65 -> [w218] mode=indexing
        tunnel: w62 -> [w217] mode=indexing
        tunnel: w60 -> [w216] mode=indexing
        tunnel: w61 -> [w215] mode=indexing
        tunnel: [w212] -> w59 mode=indexing
        n87 = for {
          tunnel: w218 -> [w222] mode=indexing
          tunnel: w217 -> [w220] mode=indexing
          tunnel: w216 -> [w221] mode=indexing
          tunnel: w215 -> [w219] mode=indexing
          tunnel: [w229] -> w214 mode=indexing
          tunnel: [w225] -> w213 mode=indexing
          w233 = "%,;%1.4f" ("format string")
          n88 = Format Value(format string=w233, value (0)=w222) -> (output string=w224:string)  [unwired: 1 in]
          n89 = Format Value(format string=w233, value (0)=w221) -> (output string=w223:string)  [unwired: 1 in]
          n90 = Select(t="", s=w220, f="*") -> (s? t:f=w230:string)
          n91 = Select(t="", s=w219, f="*") -> (s? t:f=w226:string)
          n92 = Concatenate Strings(w223, w226) -> (w225:string)
          n93 = Concatenate Strings(w224, w230) -> (w229:string)
        }
        n94 = Build Array (concatenate)(w214, w213) -> (w212:string[])
      }
      n95 = call "REPORT.BIN TO STRING.vi"("Resultado test"=w77) -> ("OK, Fault"=w35:string)  [unwired: 14 in]
      n96 = Format Into String(format string="[%d.8.1# FINAL RESULT DIGITAL OFFSET]\nDIGITAL OFFSET TEST\\t%s" ("string"), initial string=w41, w12, w35) -> (resulting string=w75:string)  [unwired: 1 in, 1 out]
      n97 = Format Value(format string="%,;%1.4f", value (0)=w68) -> (output string=w73:string)  [unwired: 1 in]
      n98 = call "REPEORT.CAMBIO LINEA.vi"("Text Out"=w75) -> ("String"=w37:string)  [unwired: 8 in]
      n99 = Build Array(w73) -> (w72:string[])
      n100 = Build Array(w72) -> (w71:string[][])
      n101 = Format Into String(format string="%d.8.2# LIMITS COMPARATION DIGITAL OFFSET TEST" ("Secction"), w12) -> (resulting string=w33:string)  [unwired: 2 in, 1 out]
      n102 = call "REPORT.Create Table.vi"("Secction"=w33, "Column Headers"=string[] ["UPPER"], "Text 2d"=w71, "Text In"=w37) -> ("Text Out"=w69:string)  [unwired: 4 in, 1 out]
      n103 = Format Into String(format string="%d.8.3# VALUES NOISE (ADC) (%.3g)" ("Secction"), w12, w9) -> (resulting string=w31:string)  [unwired: 2 in, 1 out]
      n104 = call "REPORT.Create Table.vi"("Secction"=w31, "Row Headers"=w13, "Column Headers"=w14, "Text 2d"=w59, "Text In"=w69) -> ("Text Out"=w26:string)  [unwired: 3 in, 1 out]
      n105 = Format Into String(format string="%d.8.4# VALUES DIGITAL OFFSET (ADC) (%.3g)" ("Secction"), w12, w9) -> (resulting string=w23:string)  [unwired: 2 in, 1 out]
      n106 = call "REPORT.Create Table.vi"("Secction"=w23, "Row Headers"=w13, "Column Headers"=w14, "Text 2d"=w15, "Text In"=w26) -> ("Text Out"=w25:string)  [unwired: 3 in, 1 out]
      n107 = Format Into String(format string="%d.8.5# VALUES DIGITAL OFFSET (THx ASIC START/STOP) (%.3g)" ("Secction"), w12, w9) -> (resulting string=w29:string)  [unwired: 2 in, 1 out]
      n108 = call "REPORT.Create Table.vi"("Secction"=w29, "Row Headers"=w13, "Column Headers"=w14, "Text 2d"=w58, "Text In"=w25) -> ("Text Out"=w57:string)  [unwired: 3 in, 1 out]
      n109 = call "REPEORT.CAMBIO LINEA.vi"("Text Out"=w57) -> ("String"=w80:string)  [unwired: 8 in]
    }
  }
  "Text Out" <- w6
